vi "SMU Switch Handshaking RT.vi"(4 "Source:Advanced:Source Delay":dbl=4e-05 format="%#_6p", 5 "Source:Transient Response":i32(ring)=1039 items=["Slow"=1041, "Normal"=1038, "Fast"=1039, "Custom"=1042], 7 "Measurement:Sense":i32(ring)=1009 items=["Local"=1008, "Remote"=1009], 8 "channels":string="0", 9 "Current":dbl=0.1 format="%#_6p", 10 "Voltage":dbl=0.6 format="%#_6p", 11 "resource name":refnum<k15>="SMU" caption="SMU resource name") -> (2 "R ch0":dbl=nan format="%#_8p")   [LabVIEW 2019]
uses:
  <instrlib>/niSwitch/niSwitch.llb/niSwitch Topologies.ctl
  <instrlib>/niSwitch/niSwitch.llb/niSwitch Trigger Input.ctl
  <instrlib>/niSwitch/niSwitch.llb/niSwitch Scan Advanced Output.ctl
  <instrlib>/niDCPower/nidcpower.llb/niDCPower Export Signal - Signal.ctl
  <instrlib>/niDCPower/nidcpower.llb/niDCPower Wait For Event - Event.ctl
  <instrlib>/niDCPower/nidcpower.llb/niDCPower Configure Digital Edge Start Trigger.vi
  <instrlib>/niDCPower/nidcpower.llb/niDCPower Configure Digital Edge Sequence Advance Trigger.vi
  <vilib>/ptbypt/NI_PtbyPt.lvlib
panel:
  out "R ch2":dbl=nan format="%#_8p"
  out "Waveform Chart ch2":dbl(graph)=nan
  out "standard deviation ch2":dbl=nan format="%.6p"
  out "R ch1":dbl=nan format="%#_8p"
  out "Waveform Chart ch1":dbl(graph)=nan
  out "standard deviation ch1":dbl=nan format="%.6p"
  out "Elapsed Time (ms)":u32=169
  in  "scan advanced output (External)":T1=enum."TTL1" caption="Scan Advanced Destination"
  in  "Trigger Source":T2=enum."TTL0"
  in  "topology name":T3="2527/4-Wire 16x1 Mux" caption="Topology Name"
  in  "scan list":string="ch0:2->com0;\n\n" caption="Scan List"
  in  "resource name 2":refnum<k15>="2527" caption="Switch Resource Name"
  in  "Measurement:Aperture Time":dbl=0.0833333 format="%#_6p"
  out "error out":errorcluster={"status"=TRUE, "code"=-1074118654, "source"="niSwitch Initialize With Topology.vi<ERR>Invalid resource name.\n\nInvalid Identifier: 2527 "}
  out "current measurements":dbl[](array[numeric])
  out "voltage measurements":dbl[](array[numeric])
  in  "Measurement:Advanced:DC Noise Rejection":i32(ring)=1044 items=["Normal"=1044, "Second-Order"=1043]
  in  "Source:Advanced:Sequence Loop Count":i32=39
  out "standard deviation ch0":dbl=nan format="%.6p"
  out "Waveform Chart ch0":dbl(graph)=nan
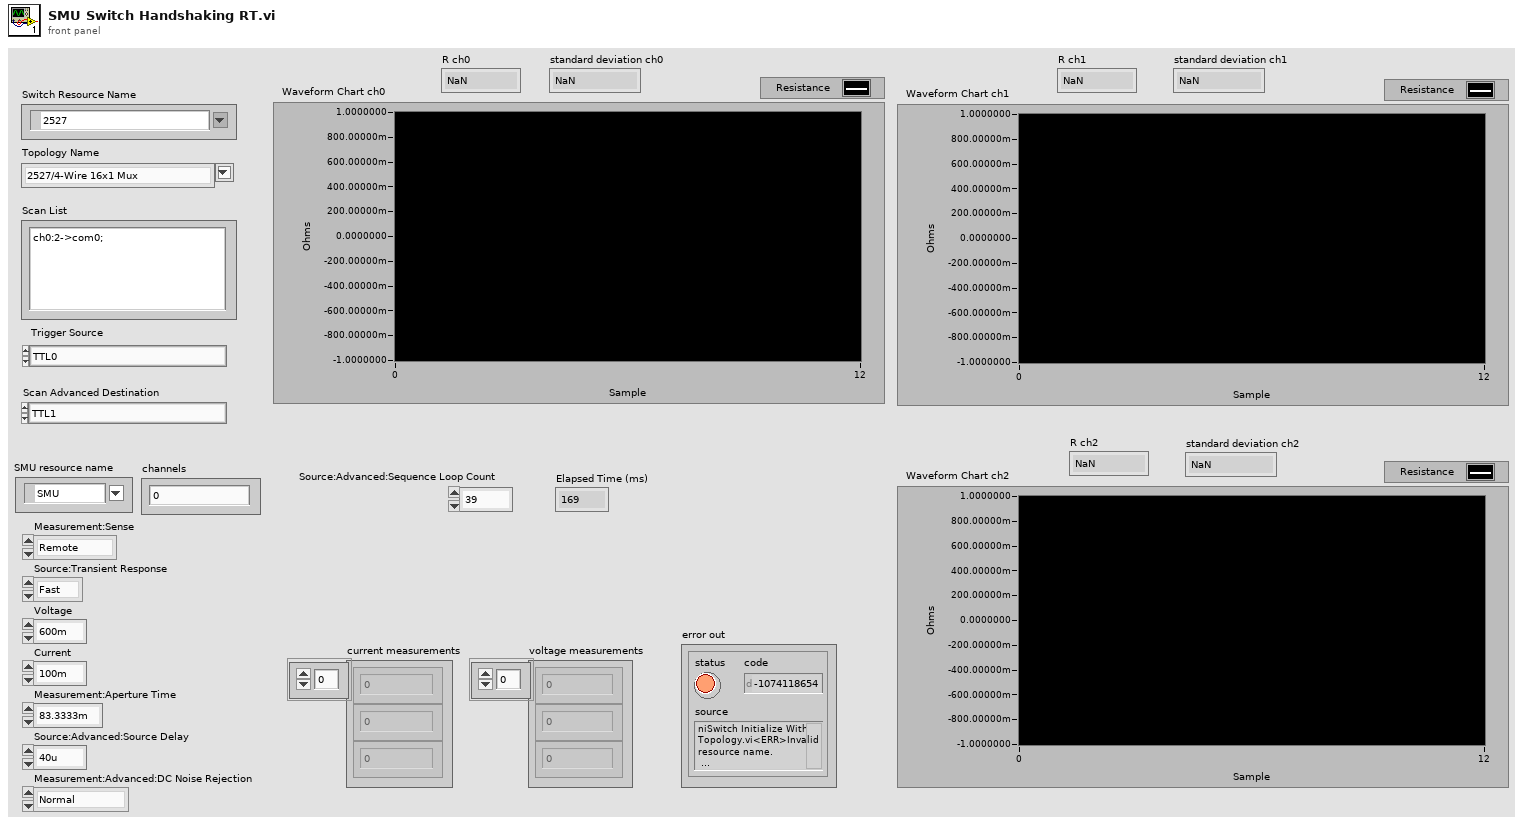
[diagram p1: front panel]
types:
  T1 = typedef "niSwitch Scan Advanced Output.ctl" = enum16{"None", "External", "TTL0", "TTL1", "TTL2", "TTL3", "TTL4", "TTL5", "TTL6", "TTL7", "ECL0", "ECL1", "PXI Star", "Rear Connector", "Front Connector", "Rear Connector Module 1", "Rear Connector Module 2", "Rear Connector Module 3", "Rear Connector Module 4", "Rear Connector Module 5", "Rear Connector Module 6", "Rear Connector Module 7", "Rear Connector Module 8", "Rear Connector Module 9", "Rear Connector Module 10", "Rear Connector Module 11", "Rear Connector Module 12", "Front Connector Module 1", "Front Connector Module 2", "Front Connector Module 3", "Front Connector Module 4", "Front Connector Module 5", "Front Connector Module 6", "Front Connector Module 7", "Front Connector Module 8", "Front Connector Module 9", "Front Connector Module 10", "Front Connector Module 11", "Front Connector Module 12"}
  T2 = typedef "niSwitch Trigger Input.ctl" = enum16{"Immediate", "External", "TTL0", "TTL1", "TTL2", "TTL3", "TTL4", "TTL5", "TTL6", "TTL7", "ECL0", "ECL1", "PXI Star", "Software Trigger Function", "Rear Connector", "Front Connector", "Rear Connector of Module 1", "Rear Connector of Module 2", "Rear Connector of Module 3", "Rear Connector of Module 4", "Rear Connector of Module 5", "Rear Connector of Module 6", "Rear Connector of Module 7", "Rear Connector of Module 8", "Rear Connector of Module 9", "Rear Connector of Module 10", "Rear Connector of Module 11", "Rear Connector of Module 12", "Front Connector of Module 1", "Front Connector of Module 2", "Front Connector of Module 3", "Front Connector of Module 4", "Front Connector of Module 5", "Front Connector of Module 6", "Front Connector of Module 7", "Front Connector of Module 8", "Front Connector of Module 9", "Front Connector of Module 10", "Front Connector of Module 11", "Front Connector of Module 12"}
  T3 = typedef "niSwitch Topologies.ctl" = string
  T4 = typedef "niDCPower Export Signal - Signal.ctl" = i32
  T5 = typedef "niDCPower Wait For Event - Event.ctl" = i32
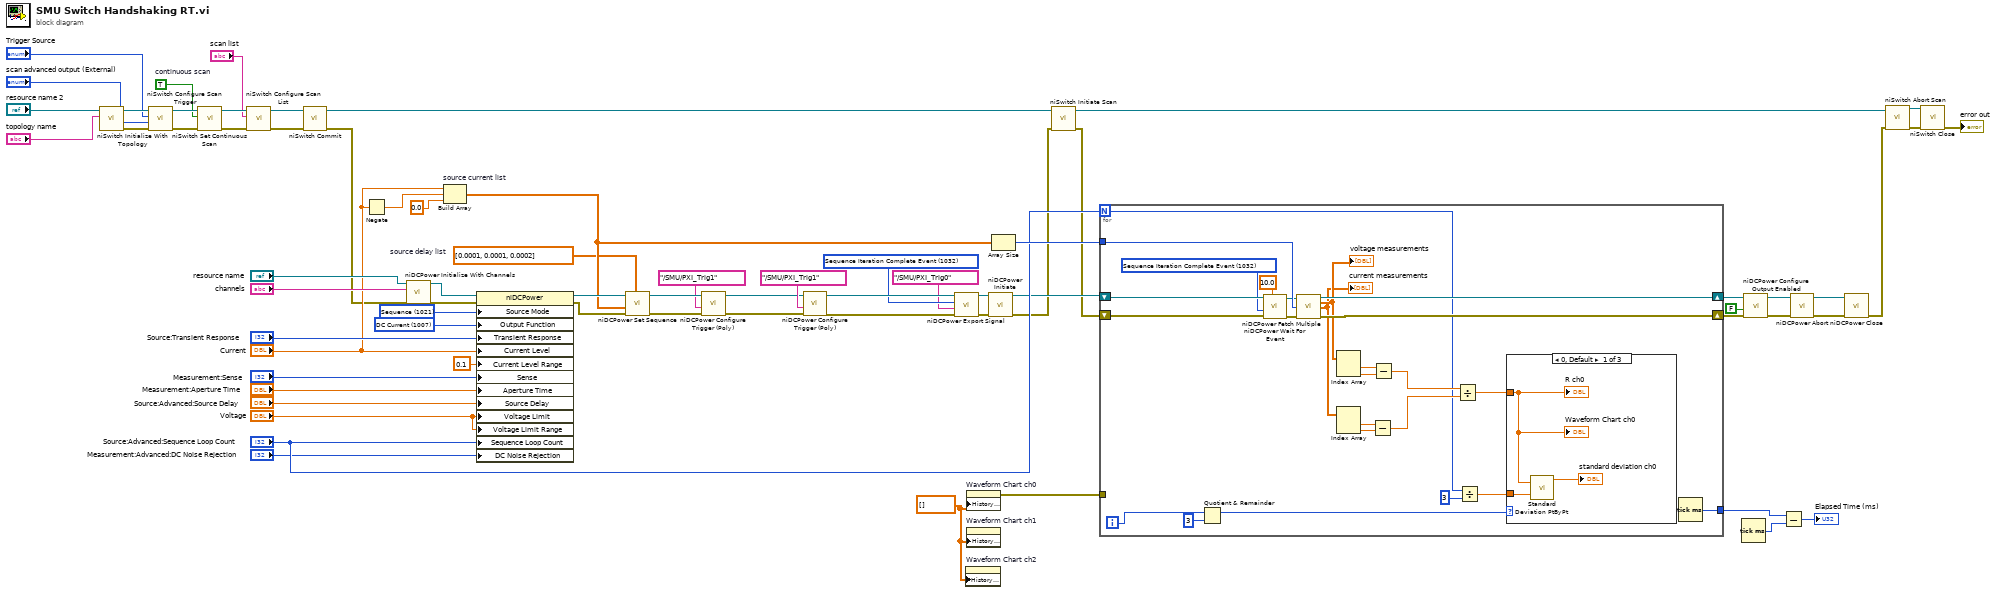
[diagram p0: block diagram]
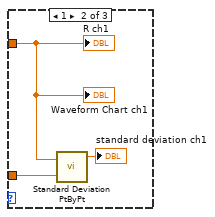
[diagram p2: hidden frame]
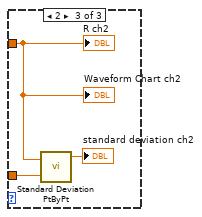
[diagram p3: hidden frame]
diagram:
  w9 = T4 1032 items=["Source Complete Event"=1030, "Measure Complete Event"=1031, "Sequence Iteration Complete Event"=1032, "Sequence Engine Done Event"=1033, "Pulse Complete Event"=1051, "Ready For Pulse Trigger Event"=1052, "Start Trigger"=1034, "Source Trigger"=1035, "Measure Trigger"=1036, "Sequence Advance Trigger"=1037, "Pulse Trigger"=1053] ("signal")
  w37 = TRUE  # continuous scan
  w43 = dbl[] [0.0001, 0.0001, 0.0002]  # source delay list
  w2 = dbl[] [] ("History Data")
  w69 = 1007 items=["DC Voltage"=1006, "DC Current"=1007, "Pulse Voltage"=1049, "Pulse Current"=1050] ("Source:Output Function")
  w70 = 1021 items=["Single Point"=1020, "Sequence"=1021] ("Source:Source Mode")
  n1 = call <instrlib>:"niSwitch Initialize With Topology.vi"("topology name"="topology name", "resource name"="resource name 2") -> ("error out"=w34:errorcluster, "instrument handle out"=w35:refnum<k15>)  [unwired: 3 in, 5 out]
  n2 = call <instrlib>:"niSwitch Configure Scan Trigger.vi"("error in (no error)"=w34, "scan advanced output (External)"="scan advanced output (External)", "trigger input (External)"="Trigger Source", "instrument handle"=w35) -> ("error out"=w38:errorcluster, "instrument handle out"=w40:refnum<k15>)  [unwired: 1 in, 5 out]
  n3 = call <instrlib>:"niSwitch Set Continuous Scan.vi"("error in (no error)"=w38, "continuous scan (False)"=w37, "instrument handle"=w40) -> ("error out"=w32:errorcluster, "instrument handle out"=w33:refnum<k15>)  [unwired: 7 out]
  n4 = call <instrlib>:"niSwitch Configure Scan List.vi"("error in (no error)"=w32, "scan list"="scan list", "instrument handle"=w33) -> ("error out"=w29:errorcluster, "instrument handle out"=w28:refnum<k15>)  [unwired: 1 in, 6 out]
  n5 = call <instrlib>:"niSwitch Commit.vi"("error in (no error)"=w29, "instrument handle"=w28) -> ("error out"=w23:errorcluster, "instrument handle out"=w27:refnum<k15>)  [unwired: 8 out]
  n6 = Negate(x="Current") -> (-x=w62:dbl)
  n7 = call <instrlib>:"niDCPower Initialize With Channels.vi"("error in (no error)"=w23, "channels"="channels", "resource name"="resource name") -> ("error out"=w57:errorcluster, "instrument handle out"=w58:refnum<k15>)  [unwired: 7 in]
  n8 = Build Array "source current list"("Current", w62, 0.0 ("element")) -> (w61:dbl[])
  n9 = property class="niDCPower"(reference=w58, error in=w57, "Source Mode"=w70, "Output Function"=w69, "Transient Response"="Source:Transient Response", "Current Level"="Current", "Current Level Range"=0.1 ("Source:DC Current:Current Level Range"), "Sense"="Measurement:Sense", "Aperture Time"="Measurement:Aperture Time", "Source Delay"="Source:Advanced:Source Delay", "Voltage Limit"="Voltage", "Voltage Limit Range"="Voltage", "Sequence Loop Count"="Source:Advanced:Sequence Loop Count", "DC Noise Rejection"="Measurement:Advanced:DC Noise Rejection") -> (reference out=w65:refnum<k15>, error out=w66:errorcluster)
  n10 = call <instrlib>:"niDCPower Set Sequence.vi"("source delays"=w43, "error in (no error)"=w66, "values"=w61, "instrument handle"=w65) -> ("error out"=w17:errorcluster, "instrument handle out"=w18:refnum<k15>)  [unwired: 6 in]
  n11 = call-poly <instrlib>:"niDCPower Configure Trigger (Poly).vi"("error in (no error)"=w17, "input terminal"=tag "/SMU/PXI_Trig1", "instrument handle"=w18) -> ("error out"=w13:errorcluster, "instrument handle out"=w14:refnum<k15>)  [unwired: 7 in]
  n12 = call-poly <instrlib>:"niDCPower Configure Trigger (Poly).vi"("error in (no error)"=w13, "input terminal"=tag "/SMU/PXI_Trig1", "instrument handle"=w14) -> ("error out"=w8:errorcluster, "instrument handle out"=w10:refnum<k15>)  [unwired: 7 in]
  n13 = call <instrlib>:"niDCPower Export Signal.vi"("error in (no error)"=w8, "output terminal"=tag "/SMU/PXI_Trig0", "signal"=w9, "instrument handle"=w10) -> ("error out"=w11:errorcluster, "instrument handle out"=w12:refnum<k15>)  [unwired: 6 in]
  n14 = property on="Waveform Chart ch2" class="WFChart (strict)"("History Data"=w2) -> ()  [unwired: 2 in, 2 out]
  n15 = property on="Waveform Chart ch0" class="WFChart (strict)"("History Data"=w2) -> (error out=w52:errorcluster)  [unwired: 2 in, 1 out]
  n16 = property on="Waveform Chart ch1" class="WFChart (strict)"("History Data"=w2) -> ()  [unwired: 2 in, 2 out]
  n17 = call <instrlib>:"niDCPower Initiate.vi"("error in (no error)"=w11, "instrument handle"=w12) -> ("error out"=w22:errorcluster, "instrument handle out"=w41:refnum<k15>)  [unwired: 8 in]
  n18 = Array Size(array=w61) -> (size(s)=w63:i32)
  n19 = call <instrlib>:"niSwitch Initiate Scan.vi"("error in (no error)"=w22, "instrument handle"=w27) -> ("error out"=w21:errorcluster, "instrument handle out"=w30:refnum<k15>)  [unwired: 8 out]
  n20 = for {
    N: "Source:Advanced:Sequence Loop Count" -> [w73]
    tunnel: w63 -> [w95]
    shift-right: [w87] -> w48
    shift-left: w21 -> [w94]
    shift-right: [w88] -> w49
    shift-left: w41 -> [w93]
    tunnel: w52 -> [_]
    tunnel: [w77] -> w6
    i -> [w76]
    w92 = T5 1032 items=["Source Complete Event"=1030, "Measure Complete Event"=1031, "Sequence Iteration Complete Event"=1032, "Sequence Engine Done Event"=1033, "Pulse Complete Event"=1051, "Ready For Pulse Trigger Event"=1052] ("event")
    n21 = Quotient & Remainder(x=w76, y=3) -> (x-y*floor(x/y)=w74:i32)  [unwired: 1 out]
    n22 = call <instrlib>:"niDCPower Wait For Event.vi"("timeout (sec)"=10.0, "error in (no error)"=w94, "event"=w92, "instrument handle"=w93) -> ("error out"=w89:errorcluster, "instrument handle out"=w90:refnum<k15>)  [unwired: 6 in]
    n23 = call <instrlib>:"niDCPower Fetch Multiple.vi"("instrument handle"=w90, "count (1)"=w95, "error in (no error)"=w89) -> ("instrument handle out"=w88:refnum<k15>, "voltage measurements"=w86:dbl[], "current measurements"=w85:dbl[], "error out"=w87:errorcluster)  [unwired: 7 in, 2 out]
    "voltage measurements" <- w86
    "current measurements" <- w85
    n24 = Index Array(array=w86) -> (element #1=w84:dbl, element #2=w83:dbl)  [unwired: 2 in]
    n25 = Index Array(array=w85) -> (element #1=w81:dbl, element #2=w82:dbl)  [unwired: 2 in]
    n26 = Subtract(x=w81, y=w82) -> (x-y=w79:dbl)
    n27 = Subtract(x=w84, y=w83) -> (x-y=w80:dbl)
    n28 = Divide(x=w80, y=w79) -> (x/y=w78:dbl)
    n29 = Divide(x=w73, y=3) -> (x/y=w71:dbl)
    n30 = case shown="0, Default" w74 {
      tunnel: w78 -> [w97 w101 w103]
      tunnel: w71 -> [w98 w100 w104]
      frame 0, Default {
        n31 = call <vilib>:"Standard Deviation PtByPt.vi"("x"=w97, "sample length"=w98) -> ("standard deviation"=→"standard deviation ch0":dbl)  [unwired: 1 in, 2 out]
        "R ch0" <- w97
        "Waveform Chart ch0" <- w97
      }
      frame 1 {
        n32 = call <vilib>:"Standard Deviation PtByPt.vi"("x"=w101, "sample length"=w100) -> ("standard deviation"=→"standard deviation ch1":dbl)  [unwired: 1 in, 2 out]
        "R ch1" <- w101
        "Waveform Chart ch1" <- w101
      }
      frame 2 {
        n33 = call <vilib>:"Standard Deviation PtByPt.vi"("x"=w103, "sample length"=w104) -> ("standard deviation"=→"standard deviation ch2":dbl)  [unwired: 1 in, 2 out]
        "R ch2" <- w103
        "Waveform Chart ch2" <- w103
      }
    }
    n34 = Tick Count (ms)() -> (millisecond timer value=w77:u32)
  }
  n35 = Tick Count (ms)() -> (millisecond timer value=w5:u32)
  n36 = call <instrlib>:"niDCPower Configure Output Enabled.vi"("error in (no error)"=w48, "output enabled"=FALSE, "instrument handle"=w49) -> ("error out"=w51:errorcluster, "instrument handle out"=w50:refnum<k15>)  [unwired: 7 in]
  n37 = Subtract(x=w6, y=w5) -> (x-y=→"Elapsed Time (ms)":u32)
  n38 = call <instrlib>:"niDCPower Abort.vi"("error in (no error)"=w51, "instrument handle"=w50) -> ("error out"=w60:errorcluster, "instrument handle out"=w59:refnum<k15>)  [unwired: 8 in]
  n39 = call <instrlib>:"niDCPower Close.vi"("error in (no error)"=w60, "instrument handle"=w59) -> ("error out"=w20:errorcluster)  [unwired: 9 in]
  n40 = call <instrlib>:"niSwitch Abort Scan.vi"("error in (no error)"=w20, "instrument handle"=w30) -> ("error out"=w36:errorcluster, "instrument handle out"=w39:refnum<k15>)  [unwired: 8 out]
  n41 = call <instrlib>:"niSwitch Close.vi"("error in (no error)"=w36, "instrument handle"=w39) -> ("error out"=→"error out":errorcluster)  [unwired: 9 out]
